vi "Recursive Remove Contained Empty Folders.vi"(8 "error in (no error)":errorcluster, 11 "Path":path) -> (0 "error out":errorcluster)   [LabVIEW 2017]
doc: "Deletes every empty folder below Path, working from the deepest level upwards so folders that only become empty are removed as well."
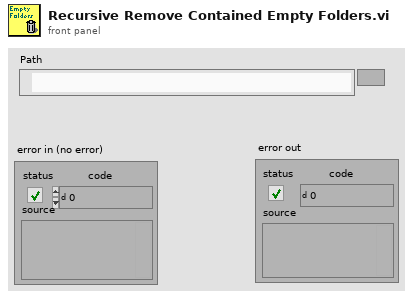
[diagram p1: front panel]
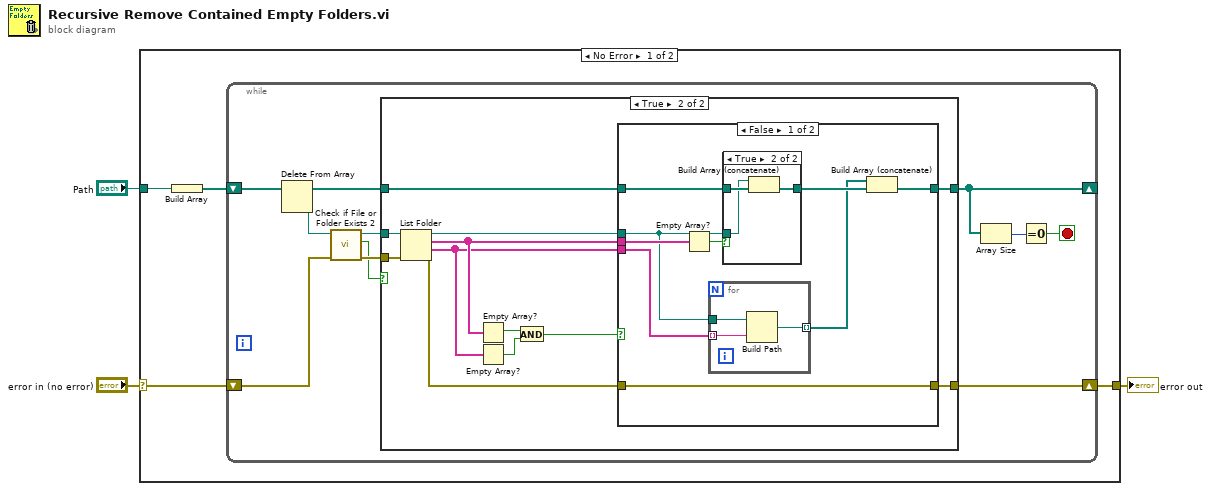
[diagram p0: block diagram]
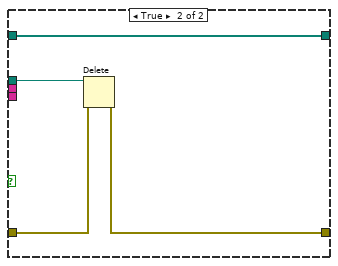
[diagram p4: hidden frame]
diagram:
  n1 = case shown="No Error" "error in (no error)" {
    selector: "error in (no error)" -> [w4 w53]
    tunnel: "Path" -> [w7 _]
    tunnel: [w5 w53] -> w2
    frame No Error {
      n2 = Build Array(w7) -> (w6:path[])
      n3 = while {
        shift-right: [w13] -> _
        shift-left: w6 -> [w18]
        shift-right: [w14] -> w5
        shift-left: w4 -> [w9]
        stop <- w15 stop-if-true
        n4 = Delete From Array(array=w18) -> (deleted portion=w17:path, array with subset deleted=w12:path[])  [unwired: 2 in]
        n5 = call "Check if File or Folder Exists 2.vi"("error in (no error)"=w9, "path"=w17) -> ("error out"=w10:errorcluster, "file or folder exists?"=w8:bool, "dup path"=w11:path)  [unwired: 7 in]
        n6 = case shown="True" w8 {
          tunnel: [w19 w30] -> w14
          tunnel: [w20 w27] -> w13
          tunnel: w12 -> [w20 w26]
          tunnel: w11 -> [_ w22]
          tunnel: w10 -> [w19 w21]
          frame False {
          }
          frame True {
            n7 = List Folder(path=w22, error in=w21) -> (path out=w31:path, filenames=w25:string[], folder names=w24:string[], error out=w23:errorcluster)  [unwired: 2 in]
            n8 = Empty Array?(array=w25) -> (empty?=w28:bool)
            n9 = Empty Array?(array=w24) -> (empty?=w32:bool)
            n10 = And(x=w28, y=w32) -> (x .and. y?=w29:bool)
            n11 = case shown="False" w29 {
              tunnel: w31 -> [w35 w52]
              tunnel: [w33 w51] -> w30
              tunnel: [w37 w50] -> w27
              tunnel: w26 -> [w40 w50]
              tunnel: w25 -> [w41 _]
              tunnel: w24 -> [w36 _]
              tunnel: w23 -> [w33 w49]
              frame False {
                n12 = Empty Array?(array=w41) -> (empty?=w39:bool)
                n13 = for {
                  tunnel: w36 -> [w44] mode=indexing
                  tunnel: w35 -> [w43]
                  tunnel: [w42] -> w34 mode=indexing
                  n14 = Build Path(base path=w43, name or relative path=w44) -> (appended path=w42:path)
                }
                n15 = case shown="True" w39 {
                  tunnel: w40 -> [w45 w48]
                  tunnel: [w45 w47] -> w38
                  tunnel: w35 -> [_ w46]
                  frame False {
                  }
                  frame True {
                    n16 = Build Array (concatenate)(w46, w48) -> (w47:path[])
                  }
                }
                n17 = Build Array (concatenate)(w34, w38) -> (w37:path[])
              }
              frame True {
                n18 = Delete(path (use dialog)=w52, error in=w49) -> (error out=w51:errorcluster)  [unwired: 3 in, 2 out]
              }
            }
          }
        }
        n19 = Array Size(array=w13) -> (size(s)=w16:i32)
        n20 = Equal To 0?(x=w16) -> (x = 0?=w15:bool)
      }
    }
    frame Error {
    }
  }
  "error out" <- w2
